vi "Initialize Stage.vi"(11 "Automation Refnum in":refnum<k7>(container)) -> (0 "error out":errorcluster, 3 "reference out":refnum<k7>)   [LabVIEW 2020, in "Rotation Stage.lvlib"]
uses:
  Rotation Stage.lvlib
  <vilib>/Utility/config.llb/Read Key (I32).vi
  <vilib>/Utility/config.llb/NI_LVConfig.lvlib
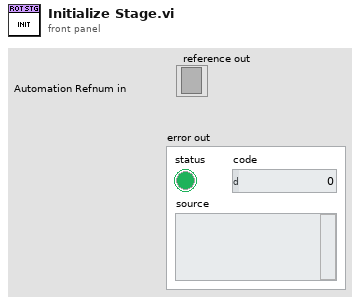
[diagram p1: front panel]
types:
  T1 = typedef "NI_LVConfig.lvlib/Config Data RefNum.ctl" = refnum<k1>
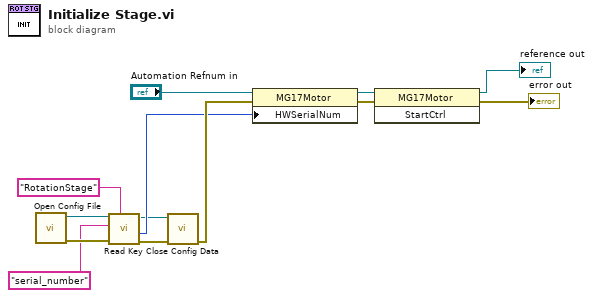
[diagram p0: block diagram]
diagram:
  n1 = call "Open Config File.vi"() -> ("error out"=w11:errorcluster, "Refnum out"=w7:T1)  [unwired: 10 in]
  n2 = call-poly <vilib>:"Read Key.vi"("section"="RotationStage", "error in (no error)"=w11, "key"="serial_number", "refnum"=w7) -> ("error out"=w12:errorcluster, "value"=w8:i32, "refnum out"=w6:T1)  [unwired: 4 in, 1 out]
  n3 = call <vilib>:"Close Config Data.vi"("error in (no error)"=w12, "refnum"=w6) -> ("error out"=w13:errorcluster)  [unwired: 8 in, 1 out]
  n4 = property class="MG17Motor"(reference="Automation Refnum in", error in=w13, "HWSerialNum"=w8) -> (reference out=w3:refnum<k7>, error out=w4:errorcluster)
  n5 = invoke class="MG17Motor" method="StartCtrl"(reference=w3, error in=w4) -> (reference out=→"reference out":refnum<k7>, error out=→"error out":errorcluster)  [unwired: 1 in, 1 out]
